vi "Compressor With Cylinder 2.vi"() -> ()   [LabVIEW 2019]
doc: "Compressor with Cylinder \n\nThis example shows how to control a compressor, extend and retract a cylinder, and optionally use a limit switch to retract automatically.\n\nThis example works with the PCM (Pneumatic Control Module) communicating with the roboRIO over CAN bus. The PCM must also be supplied with 12V DC from the PDP (Power Distribution Panel).\n\nThe Compressor, Pressure Switch, and Solenoids are all wired to the PCM \n\nThe Limit Switch is wired to DIO 9. It causes the cylinder to retract when the Auto Retract button is pressed.\n\nRefer to the Pneumatics Manual for air connections. Your pneumatics setup should include a compressor, pressure switch, tank, regulator, valve, flow controls, cylinder, plug valve, etc.\n\nTo run this example you should have a pneumatic system with air pressure connected to the P input on the SMC double solenoid valve. The A output of the valve should be connected via a flow control to the backend of a cylinder. The B output of the valve should be connected via a flow control to the frontend of a cylinder. When the cylinder is extended, it should physically depress the Limit Switch.\n\nWith the VI running, pressing the Extend button will push the cylinder shaft out, and pressing the Retract button will pull it back. Notice that the Extend and Retract buttons have their Mechanical Action set to Latch When Pressed. This means they stay pressed (ON) until they are read by the program, then they return to the OFF position. This works because once the SMC solenoid valve is pulled one direction, it stays in that position until it is pulled in the opposite direction - it only needs to be momentarily energized. The Auto Retract button can be used to make the cylinder return automatically. With the Auto Retract button ON, pressing the Extend button will push the cylinder out, and it will retract when it hits the limit switch.\n\nThis example expects a USB cable connected from your development PC to the Type B USB Jack (next to the power input) on the roboRIO.\n\nThis example expects the Driver Station to be running."
uses:
  <vilib>/Rock Robotics/SystemInterfaces/DIO/FPGA_DIOChannel.ctl
  <vilib>/Rock Robotics/WPI/Solenoid/WPI_SolenoidChannel.ctl
  <vilib>/Rock Robotics/WPI/Solenoid/WPI_SolenoidValue.ctl
  <vilib>/Rock Robotics/WPI/Solenoid/WPI_SolenoidOpenDouble.vi
  <vilib>/Rock Robotics/WPI/Utilities/WPI_GetSetVariantRefNum.vi
  <vilib>/Rock Robotics/Network Tables/NT Write Boolean Array.vi
  <vilib>/Rock Robotics/WPI/Solenoid/WPI_SolenoidSetEnum.vi
panel:
  out "Compressor Running":bool
  out "Cylinder Limit":bool
  in  "Limit Switch Channel":T1=enum."DIO 9"
  in  "Auto Retract":bool
  out "Compressor Monitoring":bool
  in  "stop":bool
  # "Set these inputs before running."
  # "roboRIO Wiring Diagram"
  # "when extended, the cylinder should depress this"
  # "Limit\nSwitch"
  # "These can be set while running."
  # "Pneumatic Control Module Wiring Diagram"
  # "Output information."
  # "Connect\nPower in\nHere"
  # "Connect\nCompressor\nHere"
  # "tubing port for retract side of cylinder"
  # "tubing port for extend side of cylinder"
  # "Pressure\nSwitch"
  # "SMC double solenoid valve"
  # "CAN"
  # "COMPRESSOR OUT"
  # "PRESSURE"
  # "NC"
  # "C"
  # "B"
  # "A"
  # "B"
  # "A"
  # "COM"
  # "NC"
  # "NO"
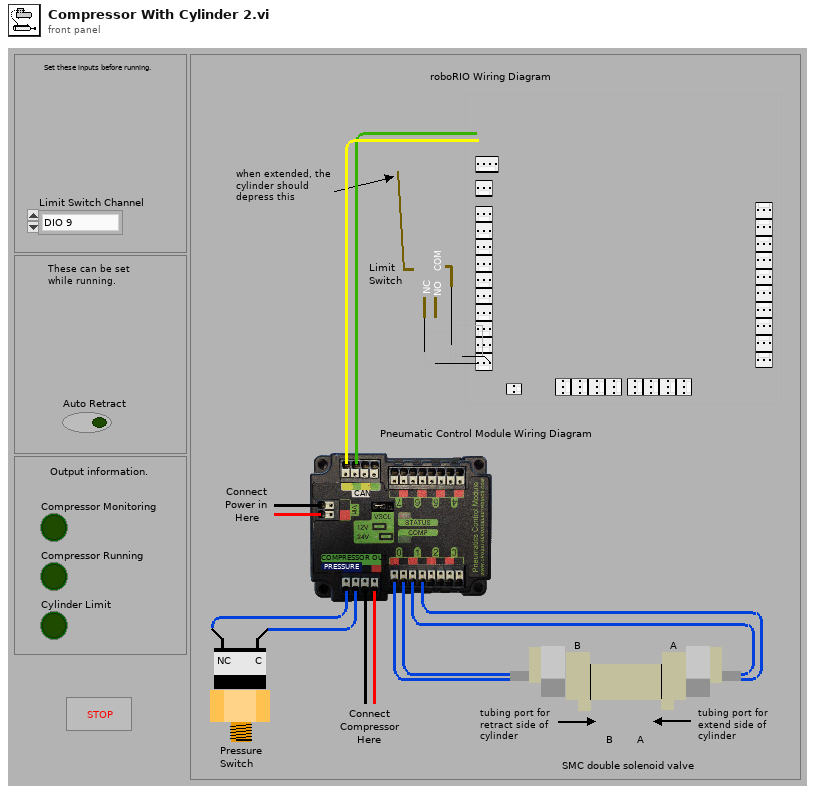
[diagram p1: front panel]
types:
  T1 = typedef "FPGA_DIOChannel.ctl" = enum8{"DIO 0", "DIO 1", "DIO 2", "DIO 3", "DIO 4", "DIO 5", "DIO 6", "DIO 7", "DIO 8", "DIO 9", "DIO MXP 0", "DIO MXP 1", "DIO MXP 2", "DIO MXP 3", "DIO MXP 4", "DIO MXP 5", "DIO MXP 6", "DIO MXP 7", "DIO MXP 8", "DIO MXP 9", "DIO MXP 10", "DIO MXP 11", "DIO MXP 12", "DIO MXP 13", "DIO MXP 14", "DIO MXP 15", "SPI Port CS1", "SPI Port CS2", "SPI Port CS3", "SPI Port MISO", "SPI Port MOSI", "Invalid"}
  T2 = typedef "WPI_SolenoidChannel.ctl" = enum8{"Solenoid 0", "Solenoid 1", "Solenoid 2", "Solenoid 3", "Solenoid 4", "Solenoid 5", "Solenoid 6", "Solenoid 7", "Invalid"}
  T3 = typedef "WPI_JoystickDevRef.ctl" = cluster{"Device":T4}
  T4 = typedef "WPI_JoystickDeviceEnum.ctl" = enum16{"USB 0", "USB 1", "USB 2", "USB 3", "USB 4", "USB 5"}
  T5 = typedef "WPI_CompressorDevRef.ctl" = cluster{"DevStatus":errorcluster, "Pneumatics Control Module":u8}
  T6 = typedef "WPI_DigitalInputDevRef.ctl" = cluster{"DevStatus":errorcluster, "DIO Channel":T1}
  T7 = typedef "WPI_SolenoidDevRef.ctl" = cluster{"DevStatus":errorcluster, "Pneumatics Control Module":u8, "Forward Solenoid Channel":T2, "Reverse Solenoid Channel":T2}
  T8 = typedef "WPI_SolenoidValue.ctl" = enum16{"Off", "On", "Forward", "Reverse"}
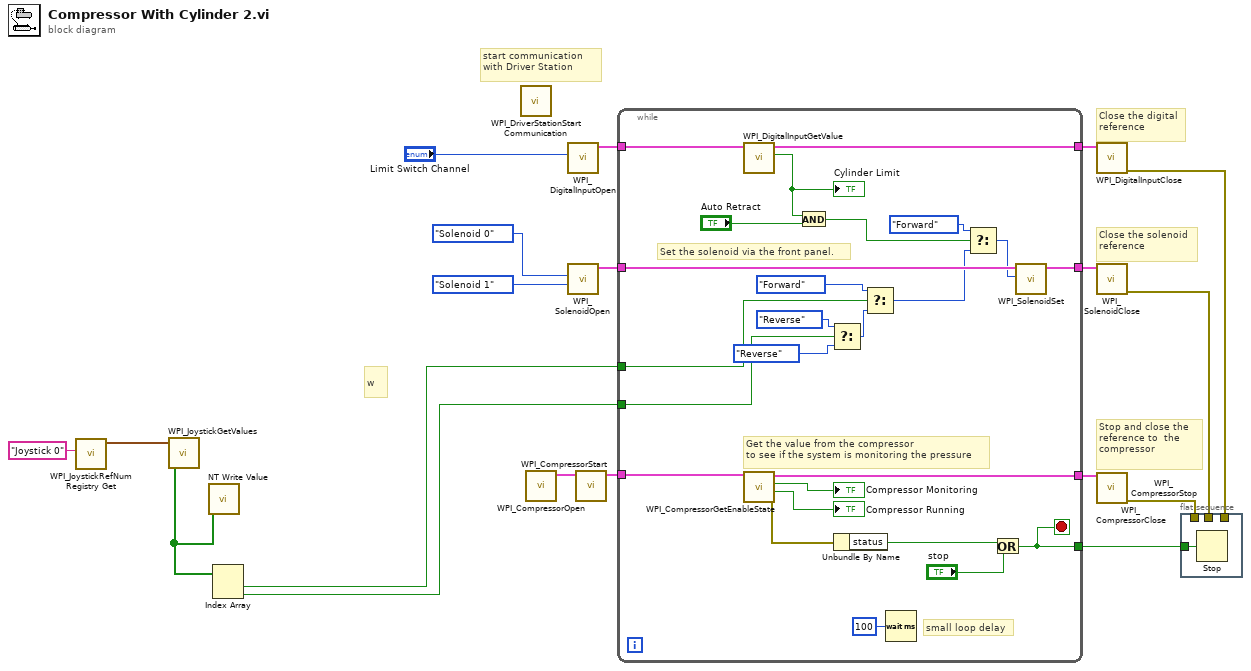
[diagram p0: block diagram]
diagram:
  # "w"
  # "Close the digital\nreference"
  # "Close the solenoid\nreference"
  # "start communication with Driver Station"
  # "Stop and close the reference to  the compressor"
  n1 = call <vilib>:"WPI_JoystickRefNum Registry Get.vi"("refnum name"="Joystick 0") -> ("JoystickDevRef"=w7:T3)  [unwired: 9 in, 1 out]
  n2 = call <vilib>:"WPI_JoystickGetValues.vi"("JoystickDevRef"=w7) -> ("Buttons"=w6:bool[])  [unwired: 6 in, 4 out]
  n3 = call-poly <vilib>:"NT Write Value.vi"("Boolean Array"=w6) -> ()  [unwired: 10 in, 1 out]
  n4 = Index Array(array=w6) -> (element #1=w3:bool, element #2=w2:bool)  [unwired: 2 in]
  n5 = call <vilib>:"WPI_DriverStationStart Communication.vi"() -> ()  [unwired: 2 in, 10 out]
  n6 = call <vilib>:"WPI_CompressorOpen.vi"() -> ("CompressorDevRef"=w12:T5)  [unwired: 14 in, 1 out]
  n7 = call <vilib>:"WPI_DigitalInputOpen.vi"("DIO Channel"="Limit Switch Channel") -> ("DigitalInputDevRef"=w15:T6)  [unwired: 1 in, 9 out]
  n8 = call-poly <vilib>:"WPI_SolenoidOpen.vi"("Reverse Solenoid Channel"=WPI_SolenoidChannel."Solenoid 1", "Forward Solenoid Channel"=WPI_SolenoidChannel."Solenoid 0") -> ("SolenoidDevRef"=w16:T7)  [unwired: 2 in, 7 out]
  n9 = call <vilib>:"WPI_CompressorStart.vi"("CompressorDevRef"=w12) -> ("CompressorDevRef"=w19:T5)  [unwired: 1 in, 9 out]
  n10 = while {
    tunnel: w19 -> [w45]
    tunnel: [w44] -> w18
    tunnel: [w42] -> w11
    tunnel: w16 -> [w37]
    tunnel: [w29] -> w17
    tunnel: w15 -> [w36]
    tunnel: [w35] -> w14
    tunnel: w3 -> [w22]
    tunnel: w2 -> [w21]
    stop <- w42 stop-if-true
    # "small loop delay"
    # "Get the value from the compressor \nto see if the system is monitoring the pressure"
    # "Set the solenoid via the front panel."
    n11 = call <vilib>:"WPI_DigitalInputGetValue.vi"("DigitalInputDevRef"=w36) -> ("Value"=w27:bool, "DigitalInputDevRef"=w35:T6)  [unwired: 1 in, 8 out]
    "Cylinder Limit" <- w27
    n12 = call <vilib>:"WPI_CompressorGetEnableState.vi"("CompressorDevRef"=w45) -> ("error out"=w40:errorcluster, "Compressor Running"=→"Compressor Running":bool, "Enabled"=→"Compressor Monitoring":bool, "CompressorDevRef"=w44:T5)  [unwired: 1 in, 6 out]
    n13 = And(x=w27, y="Auto Retract") -> (x .and. y?=w23:bool)
    n14 = Select(t=WPI_SolenoidValue."Reverse" ("Value"), s=w21, f=WPI_SolenoidValue."Reverse" ("Value")) -> (s? t:f=w31:T8)
    n15 = Unbundle By Name(w40) -> ("status"=w39:bool)
    n16 = Select(t=WPI_SolenoidValue."Forward" ("Value"), s=w22, f=w31) -> (s? t:f=w24:T8)
    n17 = Wait (ms)(milliseconds to wait=u32 100) -> ()  [unwired: 1 out]
    n18 = Select(t=WPI_SolenoidValue."Forward" ("Value"), s=w23, f=w24) -> (s? t:f=w25:T8)
    n19 = Or(x=w39, y="stop") -> (x .or. y?=w42:bool)
    n20 = call-poly <vilib>:"WPI_SolenoidSet.vi"("Value"=w25, "SolenoidDevRef"=w37) -> ("SolenoidDevRef"=w29:T7)  [unwired: 1 in, 8 out]
  }
  n21 = call <vilib>:"WPI_DigitalInputClose.vi"("DigitalInputDevRef"=w14) -> ("error out"=w8:errorcluster)  [unwired: 1 in, 9 out]
  n22 = call <vilib>:"WPI_SolenoidClose.vi"("SolenoidDevRef"=w17) -> ("error out"=w9:errorcluster)  [unwired: 1 in, 9 out]
  n23 = call <vilib>:"WPI_CompressorStop.vi"("CompressorDevRef"=w18) -> ("CompressorDevRef"=w20:T5)  [unwired: 1 in, 9 out]
  n24 = call <vilib>:"WPI_CompressorClose.vi"("CompressorDevRef"=w20) -> ("error out"=w10:errorcluster)  [unwired: 1 in, 9 out]
  n25 = flat-sequence {
    tunnel: w11 -> [w46]
    tunnel: w10 -> [_]
    tunnel: w9 -> [_]
    tunnel: w8 -> [_]
    frame #0 {
      n26 = Stop(stop? (T)=w46) -> ()
    }
  }
